vi "toXml.vi"(8 "error in (no error)":errorcluster, 11 "Delay in":refnum<class "Delay.lvclass">) -> (0 "error out":errorcluster, 2 "scriptEventXML":refnum<class "xmlNode.lvclass">, 3 "Delay out":refnum<class "Delay.lvclass">)   [LabVIEW 2011, in "Tools.lvlib" / "Scripting.lvlib" / "Delay.lvclass"]
uses:
  Delay.lvclass
  xmlNode/xmlNode.lvclass
  Delay.lvclass/Delay.ctl
  ScriptEvent.lvclass
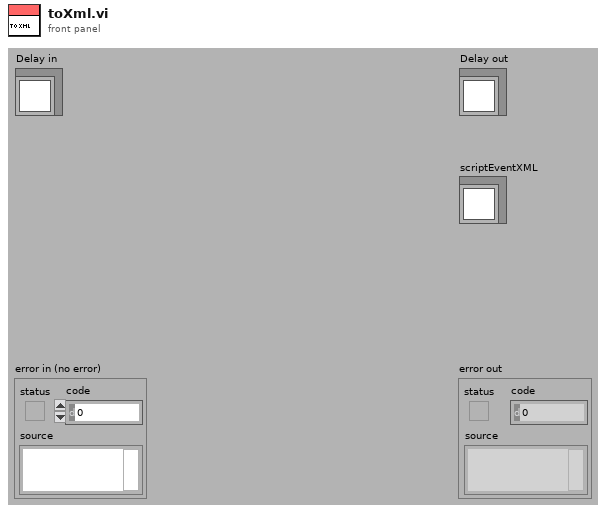
[diagram p1: front panel]
types:
  T1 = cluster{"attributeName":string, "label":string}[]
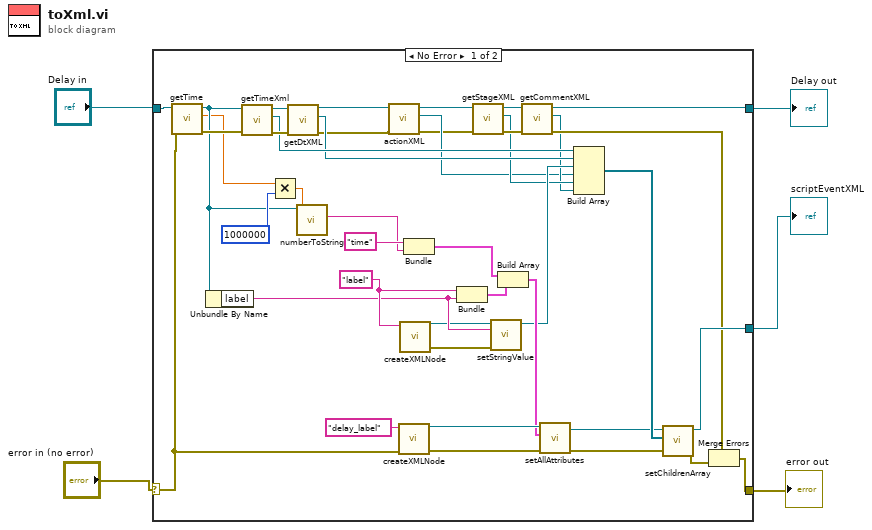
[diagram p0: block diagram]
diagram:
  n1 = case shown="No Error" "error in (no error)" {
    selector: "error in (no error)" -> [w11 w48]
    tunnel: [w34 w48] -> w3
    tunnel: [w37 w47] -> w1
    tunnel: "Delay in" -> [w21 w47]
    tunnel: [w38 _] -> w4
    frame No Error {
      w18 = "label" ("attributeName")
      n2 = call "getTime.vi"("error in (no error)"=w11, "ScriptEvent.lvclass in"=w21) -> ("error out"=w23:errorcluster, "time"=w20:dbl, "ScriptEvent.lvclass out"=w22:refnum<class "Delay.lvclass">)  [unwired: 7 in]
      n3 = Unbundle By Name(w22) -> ("label"=w17:string)
      n4 = call "getTimeXml.vi"("error in (no error)"=w23, "ScriptEvent in"=w22) -> ("error out"=w45:errorcluster, "timeXML"=w41:refnum<class "xmlNode.lvclass">, "ScriptEvent out"=w43:refnum<class "Delay.lvclass">)  [unwired: 7 in]
      n5 = Multiply(x=w20, y=1000000) -> (x*y=w25:dbl)
      n6 = call "getDtXML.vi"("error in (no error)"=w45, "ScriptEvent in"=w43) -> ("error out"=w9:errorcluster, "dtXML"=w40:refnum<class "xmlNode.lvclass">, "ScriptEvent out"=w10:refnum<class "Delay.lvclass">)  [unwired: 7 in]
      n7 = call "numberToString.vi"("Numeric"=w25, "ScriptEvent in"=w22) -> ("String"=w24:string)  [unwired: 7 in, 2 out]
      n8 = call "actionXML.vi"("error in (no error)"=w9, "ScriptEvent in"=w10) -> ("error out"=w6:errorcluster, "actionXml"=w7:refnum<class "xmlNode.lvclass">, "ScriptEvent out"=w8:refnum<class "Delay.lvclass">)  [unwired: 7 in]
      n9 = call "createXMLNode.vi"("error in (no error)"=w11, "name"="delay_label") -> ("error out"=w29:errorcluster, "xmlNode out"=w32:refnum<class "xmlNode.lvclass">)  [unwired: 8 in]
      n10 = call "createXMLNode.vi"("name"=w18) -> ("error out"=w15:errorcluster, "xmlNode out"=w16:refnum<class "xmlNode.lvclass">)  [unwired: 9 in]
      n11 = Bundle("attributeName"="time", "String"=w24) -> (w31:cluster{"attributeName":string, "String":string})  [unwired: 1 in]
      n12 = Bundle("attributeName"=w18, "label"=w17) -> (w19:cluster{"attributeName":string, "label":string})  [unwired: 1 in]
      n13 = call "getStageXML.vi"("error in (no error)"=w6, "ScriptEvent in"=w8) -> ("error out"=w44:errorcluster, "stageXML"=w13:refnum<class "xmlNode.lvclass">, "ScriptEvent out"=w42:refnum<class "Delay.lvclass">)  [unwired: 7 in]
      n14 = call-dynamic "setStringValue.vi"("error in (no error)"=w15, "stringValue"=w17, "xmlNode.lvclass in"=w16) -> ("xmlNode.lvclass out"=w14:refnum<class "xmlNode.lvclass">)  [unwired: 7 in, 1 out]
      n15 = Build Array(w31, w19) -> (w30:T1)
      n16 = call "getCommentXML.vi"("error in (no error)"=w44, "ScriptEvent in"=w42) -> ("error out"=w36:errorcluster, "commentXML"=w12:refnum<class "xmlNode.lvclass">, "ScriptEvent out"=w37:refnum<class "Delay.lvclass">)  [unwired: 7 in]
      n17 = call-dynamic "setAllAttributes.vi"("error in (no error)"=w29, "attributes"=w30, "xmlNode in"=w32) -> ("error out"=w28:errorcluster, "xmlNode out"=w27:refnum<class "xmlNode.lvclass">)  [unwired: 7 in]
      n18 = Build Array(w41, w40, w14, w7, w13, w12) -> (w39:refnum<class "xmlNode.lvclass">[])
      n19 = call-dynamic "setChildrenArray.vi"("error in (no error)"=w28, "Children"=w39, "xmlNode.lvclass in"=w27) -> ("error out"=w35:errorcluster, "xmlNode.lvclass out"=w38:refnum<class "xmlNode.lvclass">)  [unwired: 7 in]
      n20 = Merge Errors(w36, w35) -> (w34:errorcluster)
    }
    frame Error {
    }
  }
  "error out" <- w3
  "Delay out" <- w1
  "scriptEventXML" <- w4
